vi "TCP.IP Server for Ripple Detection - edited for data 3.vi"() -> ()   [LabVIEW 2021]
doc: "Demonstrates how to set up a basic TCP connection, send data to the specified port once a connection has been established, and terminate the connection once the data has been sent. This VI is designed to stop if the TCP connection is terminated. The data sent in this example is an array of random numbers."
panel:
  out "error out":errorcluster
  in  "error in (no error)":errorcluster
  out "Numeric 3":dbl
  in  "Client Closed":string="The client VI closed the connection."
  in  "Stop":bool
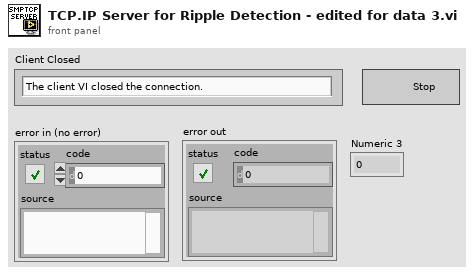
[diagram p1: front panel]
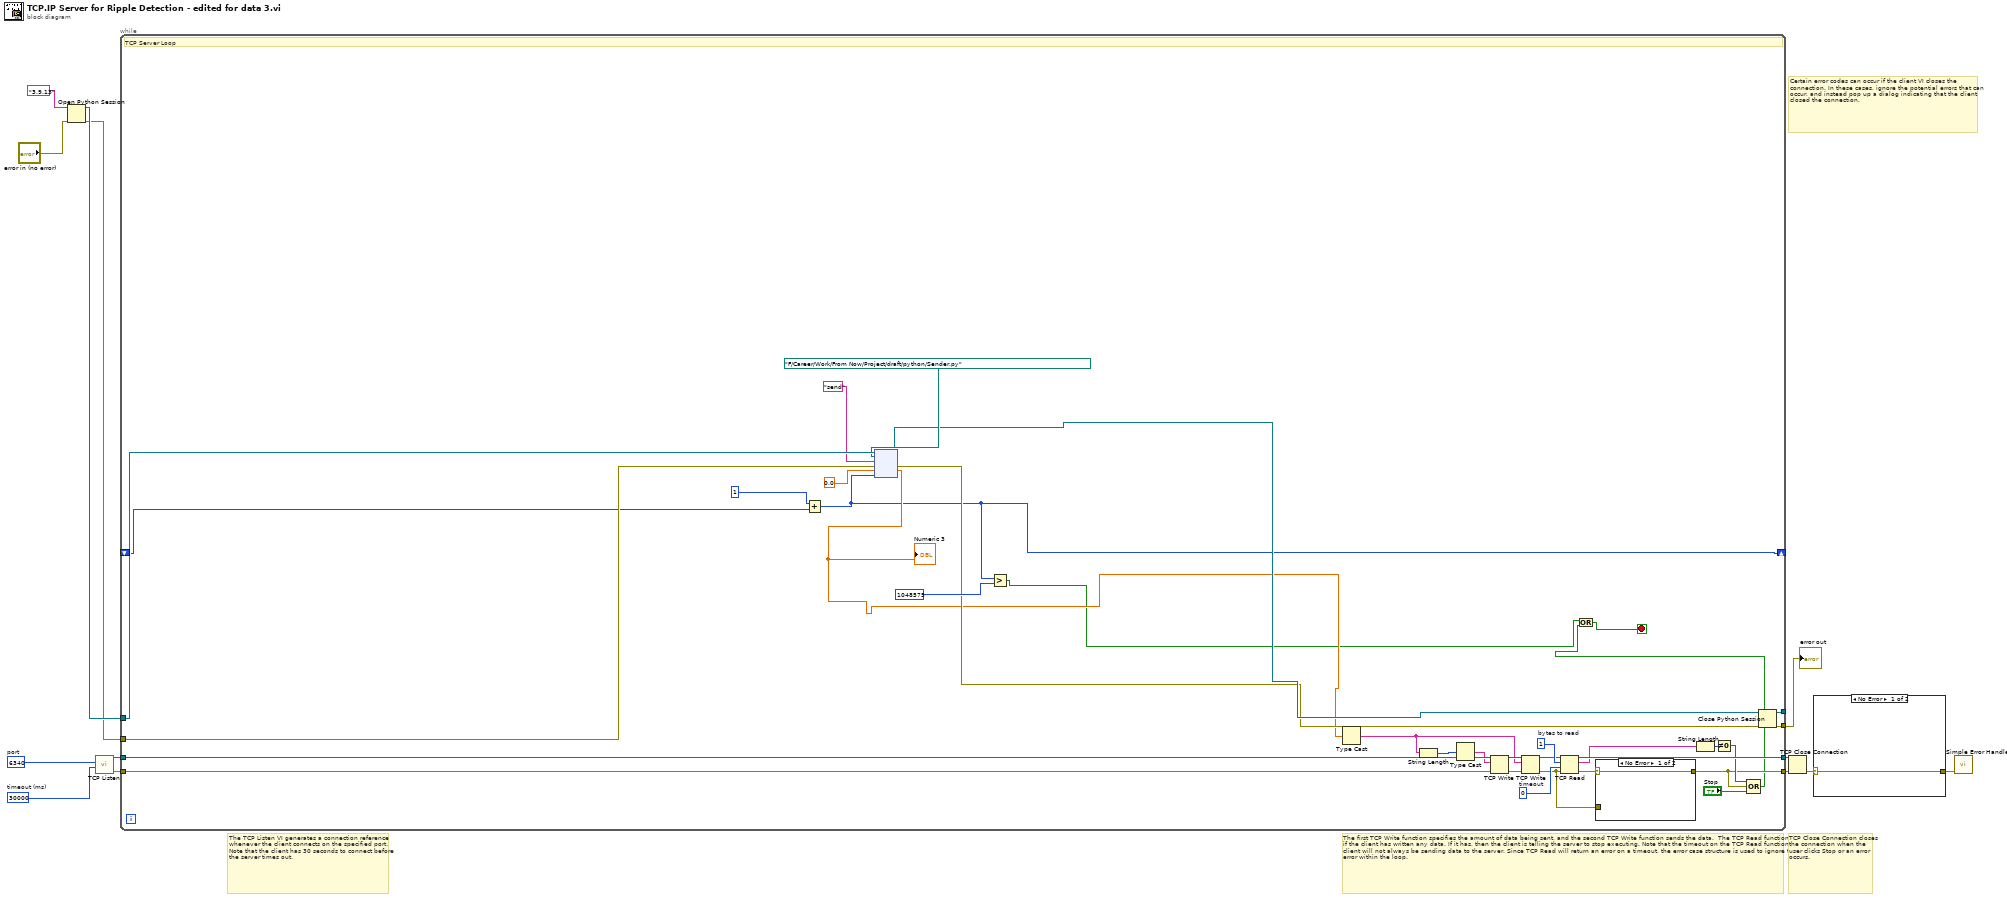
[diagram p0: block diagram]
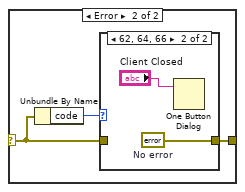
[diagram p2: hidden frame]
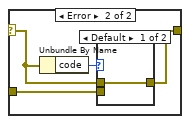
[diagram p4: hidden frame]
diagram:
  w8 = u16 6340  # port
  w9 = 30000  # timeout (ms)
  # "TCP Close Connection closes the connection when the user clicks Stop or an error occurs."
  # "The TCP Listen VI generates a connection reference whenever the client connects on the specified port. Note that the client has 30 seconds to connect before the server times out."
  # "Certain error codes can occur if the client VI closes the connection. In these cases, ignore the potential errors that can occur, and instead pop up a dialog indicating that the client closed the connection."
  # "The first TCP Write function specifies the amount of data being sent, and the second TCP Write function sends the data.  The TCP Read function checks to see if the client has written any data. If it has, then the client is telling the server to stop executing. Note that the timeout on the TCP Read function is '0', as the client will not always be sending data to the server. Since TCP Read will return an error on a timeout, the error case structure is used to ignore the timeout error within the loop."
  n1 = Open Python Session(python version="3.9.13" ("Python version"), 3:"error in (no error)") -> (session out=w6:refnum<k35>, error out=w5:errorcluster)  [unwired: 1 in]
  n2 = call <vilib>:"TCP Listen.vi"("timeout ms (wait forever: -1)"=w9, "port"=w8) -> ("error out"=w10:errorcluster, "connection ID"=w11:refnum<k5>)  [unwired: 5 in, 3 out]
  n3 = while {
    tunnel: [w32] -> w14
    tunnel: [w38] -> w15
    tunnel: w11 -> [w48]
    tunnel: w10 -> [w42]
    tunnel: w6 -> [w28]
    tunnel: w5 -> [w25]
    tunnel: [w23] -> w4
    tunnel: [w22] -> w3
    shift-right: [w19] -> _
    shift-left: _ -> [w20]
    stop <- w17 stop-if-true
    w37 = 0  # timeout
    w40 = 1  # bytes to read
    # "TCP Server Loop"
    n4 = Add(x=1, y=w20) -> (x+y=w19:i32)
    n5 = node(w28, path "F:/Career/Work/From Now/Project/draft/python/Sender.py" ("module path"), "send" ("function name"), w25, 0.0, w19) -> (w23:refnum<k35>, w22:errorcluster, w21:dbl)  [unwired: 1 in, 2 out]
    "Numeric 3" <- w21
    n6 = Greater?(x=w19, y=1048575) -> (0:w16:bool)
    n7 = Type Cast(x=w21) -> (*(type *) &x=w43:string)  [unwired: 1 out]
    n8 = String Length(string=w43) -> (length=w45:i32)
    n9 = Type Cast(x=w45) -> (*(type *) &x=w44:string)  [unwired: 1 out]
    n10 = TCP Write(connection ID=w48, data in=w44, error in (no error)=w42) -> (connection ID out=w47:refnum<k5>, error out=w46:errorcluster)  [unwired: 2 out]
    n11 = TCP Write(connection ID=w47, data in=w43, error in (no error)=w46) -> (connection ID out=w39:refnum<k5>, error out=w31:errorcluster)  [unwired: 2 out]
    n12 = TCP Read(connection ID=w39, bytes to read=w40, error in (no error)=w31, 9:w37) -> (connection ID out=w38:refnum<k5>, data out=w35:string, error out=w33:errorcluster)  [unwired: 1 out]
    n13 = case shown="No Error" w33 {
      selector: w33 -> [w49 w52]
      tunnel: [w49 w50] -> w32
      tunnel: w31 -> [_ w51]
      frame No Error {
      }
      frame Error {
        n14 = Unbundle By Name(w52) -> ("code"=w53:i32)
        n15 = case shown="Default" w53 {
          tunnel: w52 -> [w54 _]
          tunnel: w51 -> [_ w55]
          tunnel: [w54 w55] -> w50
          frame Default {
          }
          frame 56 {
          }
        }
      }
    }
    n16 = String Length(string=w35) -> (length=w36:i32)
    n17 = Not Equal To 0?(x=w36) -> (x != 0?=w34:bool)
    n18 = Compound Arithmetic op=OR(w34, w32, "Stop") -> (w18:bool)
    n19 = Or(x=w16, y=w18) -> (x .or. y?=w17:bool)
  }
  n20 = Close Python Session(session in=w4, error in=w3) -> (11:→"error out":errorcluster)
  n21 = TCP Close Connection(connection ID=w15, error in (no error)=w14) -> (error out=w13:errorcluster)  [unwired: 2 out]
  n22 = case shown="No Error" w13 {
    selector: w13 -> [w56 w58]
    tunnel: [w56 w57] -> w12
    frame No Error {
    }
    frame Error {
      n23 = Unbundle By Name(w58) -> ("code"=w59:i32)
      n24 = case shown="62, 64, 66" w59 {
        tunnel: w58 -> [w60 _]
        tunnel: [w60 w62] -> w57
        frame Default {
        }
        frame 62, 64, 66 {
          w62 = errorcluster {"status"=FALSE, "code"=0, "source"=""}  # No error
          n25 = One Button Dialog(message="Client Closed") -> ()  [unwired: 1 in, 1 out]
        }
      }
    }
  }
  n26 = call <vilib>:"Simple Error Handler.vi"("error in (no error)"=w12) -> ()  [unwired: 1 in, 8 out]
